vi "SP Calculate SYX.vi"(10 "TP Array (TXX, TXY, TYX, TYY)":cdb[](array[numeric])) -> (2 "SYX":cdb)   [LabVIEW 2011]
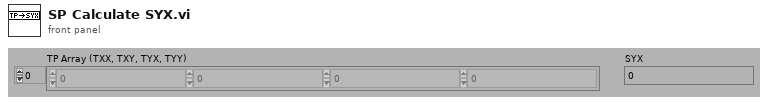
[diagram p1: front panel]
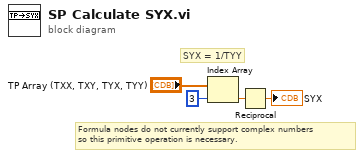
[diagram p0: block diagram]
diagram:
  # "SYX = 1/TYY"
  # "Formula nodes do not currently support complex numbers\nso this primitive operation is necessary."
  n1 = Index Array(array="TP Array (TXX, TXY, TYX, TYY)", index=3) -> (element=w2:cdb)
  n2 = Reciprocal(x=w2) -> (1/x=→"SYX":cdb)
